vi "getRamdonDate.vi"(9 "Start Day":i32=1, 10 "Action (GetDate)":enum16{"Initialize", "GetDate", "Increment Day"}(ring)=enum."GetDate") -> (2 "Ramdon date":string)   [LabVIEW 2018]
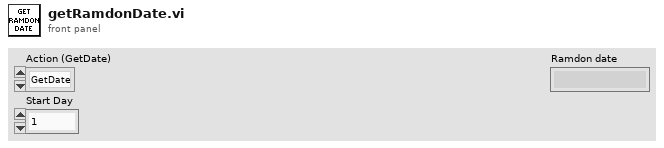
[diagram p1: front panel]
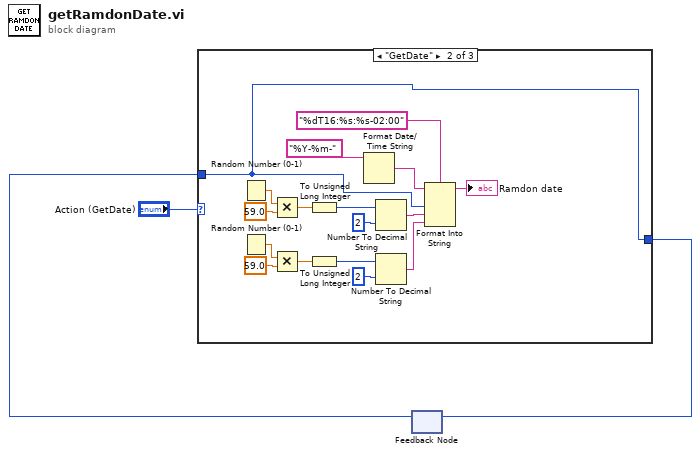
[diagram p0: block diagram]
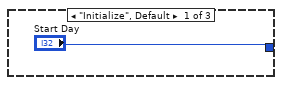
[diagram p2: hidden frame]
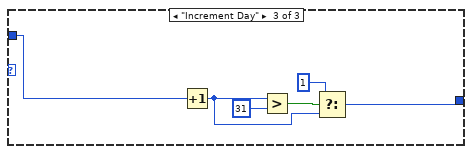
[diagram p3: hidden frame]
diagram:
  n1 = feedback #1() -> (w1:i32)  [unwired: 1 in]
  n2 = case shown="\"GetDate\"" "Action (GetDate)" {
    tunnel: ["Start Day" w5 w22] -> w2
    tunnel: w1 -> [_ w5 w23]
    frame "Initialize", Default {
    }
    frame "GetDate" {
      n3 = Random Number (0-1)() -> (number: 0 to 1=w11:dbl)
      n4 = Random Number (0-1)() -> (number: 0 to 1=w14:dbl)
      n5 = Multiply(x=w11, y=59.0) -> (x*y=w15:dbl)
      n6 = Multiply(x=w14, y=59.0) -> (x*y=w16:dbl)
      n7 = To Unsigned Long Integer(number=w15) -> (unsigned 32bit integer=w20:u32)
      n8 = To Unsigned Long Integer(number=w16) -> (unsigned 32bit integer=w18:u32)
      n9 = Format Date/Time String(time format string (%c)="%Y-%m-") -> (date/time string=w9:string)  [unwired: 2 in]
      n10 = Number To Decimal String(number=w20, width (-)=i16 2) -> (decimal integer string=w6:string)
      n11 = Number To Decimal String(number=w18, width (-)=i16 2) -> (decimal integer string=w21:string)
      n12 = Format Into String(format string="%dT16:%s:%s-02:00", initial string=w9, w5, w6, w21) -> (resulting string=→"Ramdon date":string)  [unwired: 1 in, 1 out]
    }
    frame "Increment Day" {
      n13 = Increment(x=w23) -> (x+1=w24:i32)
      n14 = Greater?(x=w24, y=31) -> (0:w26:bool)
      n15 = Select(t=1 ("y"), s=w26, f=w24) -> (s? t:f=w22:i32)
    }
  }
  n16 = feedback-in #1(w2) -> ()
